vi "Get Head Model.vi"(11 "name":string) -> (2 "function return":u32, 3 "name out":string)   [LabVIEW 2018, in "Copy of Andor SDK.lvlib"]
doc: "EXPNETTYPE unsigned int WINAPI GetHeadModel(char * name);"
uses:
  Copy of Andor SDK.lvlib
  <userlib>/Andor SDK/ATMCD32D.dll
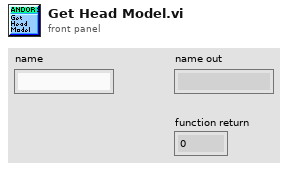
[diagram p1: front panel]
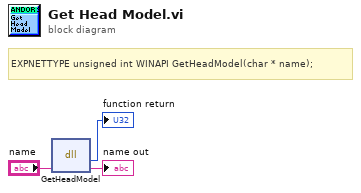
[diagram p0: block diagram]
diagram:
  # "EXPNETTYPE unsigned int WINAPI GetHeadModel(char * name);"
  n1 = dll-call lib="C:/Program Files (x86)/National Instruments/LabVIEW 2018/user.lib/Andor SDK/ATMCD32D.*" fn="GetHeadModel"("name"="name") -> (→"function return":u32, "name"=→"name out":string)  [unwired: 3 in, 2 out]
